vi "Class Object Reference..FGV.vi"(7 "FGV State":T1, 8 "error in (no error)":errorcluster, 9 "Connection Name":string, 11 "LabSFTP ref in":refnum<k24>) -> (0 "error out":errorcluster, 3 "LabSFTP ref out":refnum<k24>)   [LabVIEW 2018, in "LabSFTP.lvlib"]
doc: "<License>This software is distributed under the BSD 3-Clause License. For the full license please see license.txt or visit www.labvolution.com/license</License>"
uses:
  LabSFTP.lvlib
  FGV State..enum.ctl
  References/LabSFTP.dll
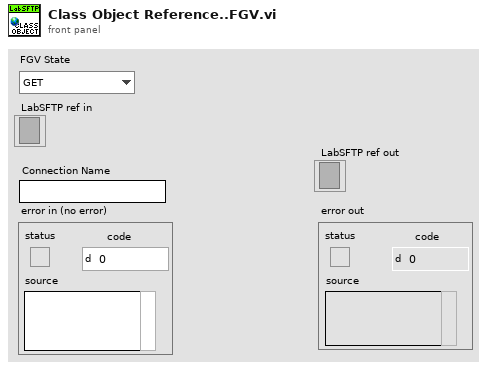
[diagram p1: front panel]
types:
  T1 = typedef "LabSFTP.lvlib/FGV State..enum.ctl" = enum16{"GET", "SET"}
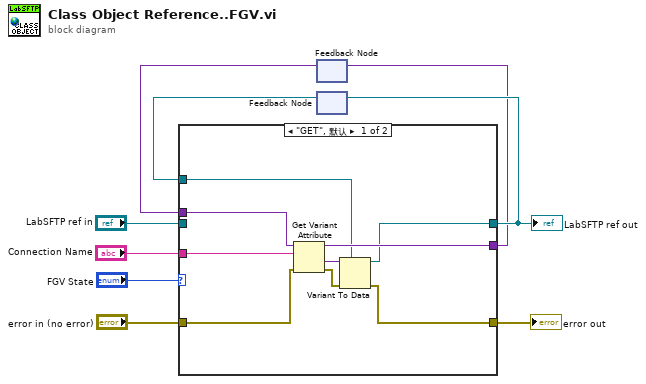
[diagram p0: block diagram]
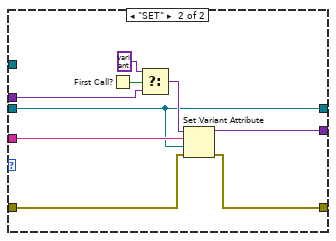
[diagram p2: hidden frame]
diagram:
  n1 = feedback #1() -> (w1:variant)  [unwired: 1 in]
  n2 = feedback #2() -> (w6:refnum<k24>)  [unwired: 1 in]
  n3 = case shown="\"GET\", 默认" "FGV State" {
    tunnel: "error in (no error)" -> [w15 w24]
    tunnel: [w14 w23] -> w8
    tunnel: "LabSFTP ref in" -> [_ w21]
    tunnel: [w11 w21] -> w4
    tunnel: w6 -> [w10 _]
    tunnel: "Connection Name" -> [w13 w22]
    tunnel: w1 -> [w16 w20]
    tunnel: [w12 w19] -> w2
    frame "GET", Default {
      n4 = Get Variant Attribute(Variant=w16, name=w13, error in=w15) -> (duplicate Variant=w12:variant, value=w17:variant, error out=w18:errorcluster)  [unwired: 1 in, 1 out]
      n5 = Variant To Data(error in=w18, type=w10, Variant=w17) -> (data=w11:refnum<k24>, error out=w14:errorcluster)
    }
    frame "SET" {
      n6 = First Call?() -> (First Call?: T/F=w26:bool)
      n7 = Select(t=variant ("variant"), s=w26, f=w20) -> (s? t:f=w27:variant)
      n8 = Set Variant Attribute(Variant=w27, name=w22, value=w21, error in=w24) -> (Variant out=w19:variant, error out=w23:errorcluster)  [unwired: 1 out]
    }
  }
  "error out" <- w8
  "LabSFTP ref out" <- w4
  n9 = feedback-in #1(w2) -> ()
  n10 = feedback-in #2(w4) -> ()
